vi "zero.vi"() -> ()   [LabVIEW 2017]
uses:
  <vilib>/myRIO/Common/Instrument Driver Framework/myRIO v1.0/DIO/typedefs/DIO Channels Enum.ctl
  <vilib>/myRIO/Common/Instrument Driver Framework/myRIO v1.0/DIO/typedefs/DIO Channels List.ctl
  <vilib>/myRIO/Common/Instrument Driver Framework/Utilities/typedefs/Generic FPGA Reference.ctl
  <vilib>/myRIO/Common/Instrument Driver Framework/Utilities/typedefs/myRIO v1.0 Reference.ctl
  <vilib>/myRIO/Common/Instrument Driver Framework/Utilities/typedefs/Hardware Version Enum.ctl
  <vilib>/myRIO/Common/Instrument Driver Framework/Utilities/typedefs/myRIO Generic Hardware Reference.ctl
  <vilib>/myRIO/Instrument Drivers/Onboard IO/DIO/typedefs/DIO Reference.ctl
  <vilib>/myRIO/Instrument Drivers/Onboard IO/DIO/DIO.lvlib
  <vilib>/myRIO/Instrument Drivers/Onboard IO/DIO/vis/Write.vi
  <vilib>/userdefined/High Color/nirio_resource_hc.ctl
  <vilib>/myRIO/Common/Instrument Driver Framework/myRIO v1.0/DIO/vis/myRIO v1.1 Open DIO.vi
  <vilib>/myRIO/Instrument Drivers/Onboard IO/DIO/vis/myRIO DIO Open.xnode
  <vilib>/myRIO/Common/Instrument Driver Framework/Utilities/vis/Is FPGA Ref Available.vi
  <vilib>/myRIO/Express VI/Onboard Devices/LED/LED Express VI.xnode
  <vilib>/myRIO/Express VI/Onboard IO/DO/DO Express VI.xnode
panel:
  in  "Array array 0-4":dbl[](array[numeric])
  out "Numeric":i32
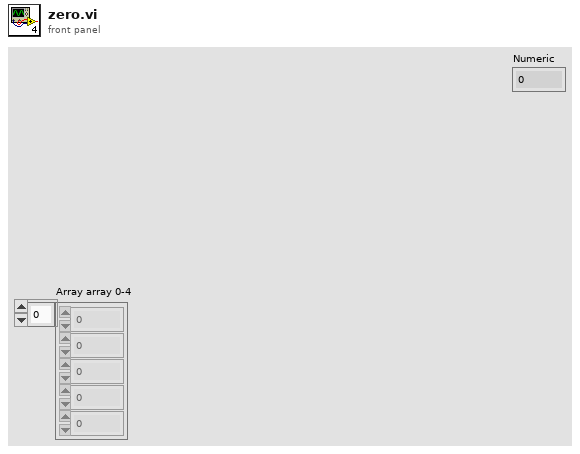
[diagram p1: front panel]
types:
  T1 = typedef "DIO.lvlib/DIO Reference.ctl" = cluster{"myRIO Reference":T2, "DIO Channels List":T6}
  T2 = typedef "myRIO Generic Hardware Reference.ctl" = cluster{"myRIO Model":T3, "myRIO Hardware Reference":T4}
  T3 = typedef "Hardware Version Enum.ctl" = enum16{"Unknown", "myRIO-1900", "myRIO-1950", "roboRIO", "NI ELVIS RIO CM"}
  T4 = typedef "myRIO v1.0 Reference.ctl" = cluster{"Generic FPGA Reference":T5, "Allow multiple opens":bool}
  T5 = typedef "Generic FPGA Reference.ctl" = refnum<k20>
  T6 = typedef "DIO Channels List.ctl" = T7[]
  T7 = typedef "DIO Channels Enum.ctl" = enum16{"Not Connected", "C/DIO0", "C/DIO1", "C/DIO2", "C/DIO3", "C/DIO4", "C/DIO5", "C/DIO6", "C/DIO7", "A/DIO0", "A/DIO1", "A/DIO2", "A/DIO3", "A/DIO4", "A/DIO5", "A/DIO6", "A/DIO7", "A/DIO8", "A/DIO9", "A/DIO10", "A/DIO11", "A/DIO12", "A/DIO13", "A/DIO14", "A/DIO15", "B/DIO0", "B/DIO1", "B/DIO2", "B/DIO3", "B/DIO4", "B/DIO5", "B/DIO6", "B/DIO7", "B/DIO8", "B/DIO9", "B/DIO10", "B/DIO11", "B/DIO12", "B/DIO13", "B/DIO14", "B/DIO15", "LED0", "LED1", "LED2", "LED3", "Button0", "DIO/DIO0", "DIO/DIO1", "DIO/DIO2", "DIO/DIO3", "DIO/DIO4", "DIO/DIO5", "DIO/DIO6", "DIO/DIO7", "DIO/DIO8", "DIO/DIO9", "SPI/CS0", "SPI/CS1", "SPI/CS2", "SPI/CS3", "LED RADIO (Green)", "LED RADIO (Red)", "LED COMM (Green)", "LED COMM (Red)", "LED MODE (Green)", "LED MODE (Red)"}
  T8 = typedef "nirio_resource_hc.ctl" = tag
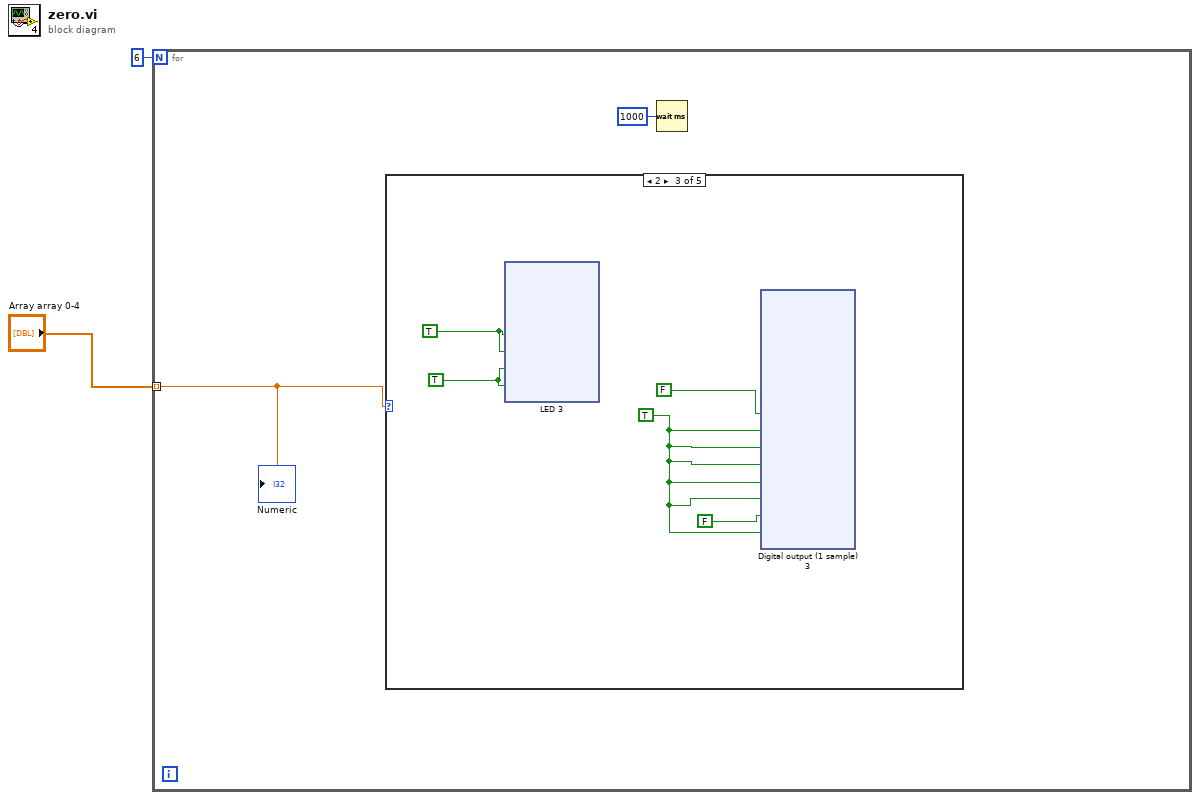
[diagram p0: block diagram]
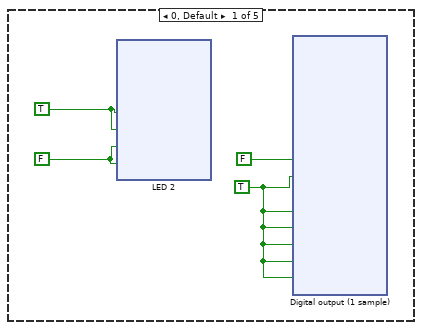
[diagram p2: hidden frame]
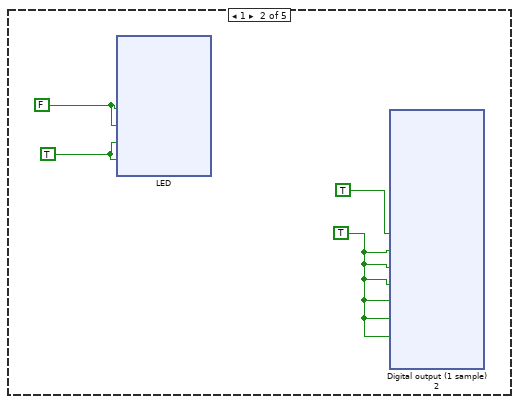
[diagram p3: hidden frame]
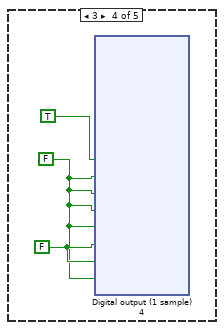
[diagram p4: hidden frame]
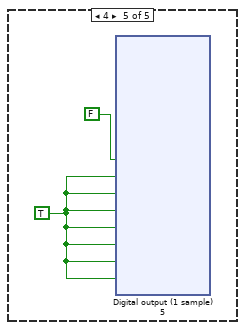
[diagram p5: hidden frame]
diagram:
  n1 = for {
    N: 6 -> [_]
    tunnel: "Array array 0-4" -> [w4] mode=indexing
    n2 = case shown="2" w4 {
      frame 0, Default {
        w5 = TRUE
        w7 = FALSE
        w8 = TRUE
        n3 = xnode "LED 2"("LED0"=w8, "LED1"=w8, "LED2"=w7, "LED3"=w7) -> ()  [unwired: 1 in, 1 out]
        n4 = xnode "Digital output (1 sample)"("A/DIO7 (Pin 25)"=FALSE, "A/DIO0 (Pin 11)"=w5, "A/DIO2 (Pin 15)"=w5, "A/DIO3 (Pin 17)"=w5, "A/DIO4 (Pin 19)"=w5, "A/DIO5 (Pin 21)"=w5, "A/DIO6 (Pin 23)"=w5) -> ()  [unwired: 2 in, 1 out]
      }
      frame 1 {
        w89 = TRUE
        w91 = TRUE
        w92 = FALSE
        n5 = xnode "LED"("LED0"=w92, "LED1"=w92, "LED2"=w91, "LED3"=w91) -> ()  [unwired: 1 in, 1 out]
        n6 = xnode "Digital output (1 sample) 2"("A/DIO7 (Pin 25)"=TRUE, "A/DIO0 (Pin 11)"=w89, "A/DIO1 (Pin 13)"=w89, "A/DIO2 (Pin 15)"=w89, "A/DIO3 (Pin 17)"=w89, "A/DIO4 (Pin 19)"=w89, "A/DIO5 (Pin 21)"=w89) -> ()  [unwired: 2 in, 1 out]
      }
      frame 2 {
        w174 = TRUE
        w176 = TRUE
        w177 = TRUE
        n7 = xnode "LED 3"("LED0"=w177, "LED1"=w177, "LED2"=w176, "LED3"=w176) -> ()  [unwired: 1 in, 1 out]
        n8 = xnode "Digital output (1 sample) 3"("A/DIO7 (Pin 25)"=FALSE, "A/DIO0 (Pin 11)"=w174, "A/DIO1 (Pin 13)"=w174, "A/DIO2 (Pin 15)"=w174, "A/DIO3 (Pin 17)"=w174, "A/DIO4 (Pin 19)"=w174, "A/DIO5 (Pin 21)"=FALSE, "A/DIO6 (Pin 23)"=w174) -> ()  [unwired: 1 in, 1 out]
      }
      frame 3 {
        w260 = FALSE ("A/DIO6 (Pin 23)")
        w259 = FALSE
        n9 = xnode "Digital output (1 sample) 4"("A/DIO7 (Pin 25)"=TRUE, "A/DIO0 (Pin 11)"=w259, "A/DIO1 (Pin 13)"=w259, "A/DIO2 (Pin 15)"=w259, "A/DIO3 (Pin 17)"=w259, "A/DIO4 (Pin 19)"=w260, "A/DIO5 (Pin 21)"=w260, "A/DIO6 (Pin 23)"=w259) -> ()  [unwired: 1 in, 1 out]
      }
      frame 4 {
        w303 = TRUE
        n10 = xnode "Digital output (1 sample) 5"("A/DIO7 (Pin 25)"=FALSE, "A/DIO0 (Pin 11)"=w303, "A/DIO1 (Pin 13)"=w303, "A/DIO2 (Pin 15)"=w303, "A/DIO3 (Pin 17)"=w303, "A/DIO4 (Pin 19)"=w303, "A/DIO5 (Pin 21)"=w303, "A/DIO6 (Pin 23)"=w303) -> ()  [unwired: 1 in, 1 out]
      }
    }
    n11 = Wait (ms)(milliseconds to wait=u32 1000) -> ()  [unwired: 1 out]
    "Numeric" <- w4
  }
